vi "read.vi"() -> ()   [LabVIEW 2013]
uses:
  <vilib>/addons/database/Connection.llb/DB Tools Open Connec (Path).vi
  <vilib>/addons/database/_DB Variant To Data/Database Variant To Data.xnode
  <vilib>/addons/database/NI_Database_API.lvlib
panel:
  out "data 3":dbl[](array[numeric])
  out "size(s)":i32
  out "values":variant[](array[variant])
  out "names":string[](array[string])
  out "type string":i16[](array[numeric])
  out "data 2":dbl[](array[numeric])
  out "Waveform Graph":dbl[](graph)
  out "data":variant[][](array[variant])
  out "error out":errorcluster
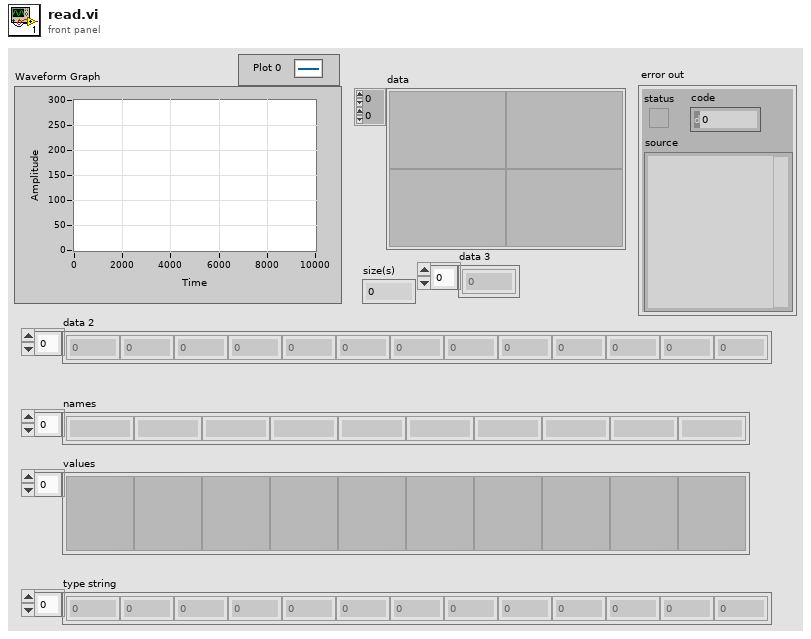
[diagram p1: front panel]
types:
  T1 = typedef "NI_Database_API.lvlib/Conn ObjectReference.ctl" = refnum<k1>
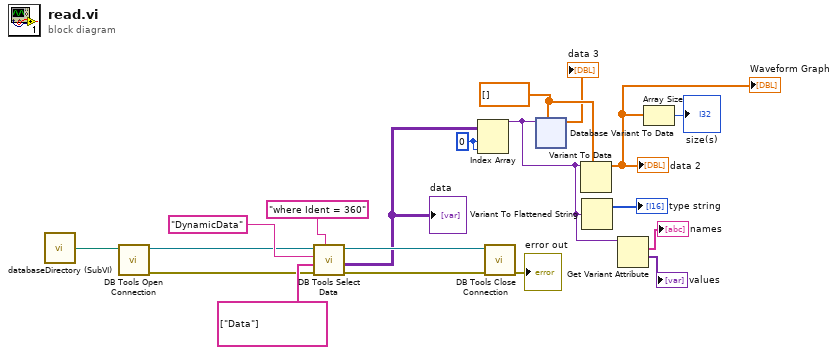
[diagram p0: block diagram]
diagram:
  w8 = dbl[] []
  w9 = 0 ("index")
  n1 = call "databaseDirectory (SubVI).vi"() -> ("Application Directory"=w14:path)  [unwired: 1 in]
  n2 = call-poly <vilib>:"DB Tools Open Connection.vi"("connection information"=w14) -> ("error out"=w13:errorcluster, "connection reference"=w12:T1)  [unwired: 7 in]
  n3 = call <vilib>:"DB Tools Select Data.vi"("condition"="where Ident = 360", "error in (no error)"=w13, "columns"=string[] ["Data"], "table"="DynamicData", "connection reference"=w12) -> ("error out"=w16:errorcluster, "data"=w10:variant[][], "connection reference out"=w17:T1)  [unwired: 1 in]
  "data" <- w10
  n4 = Index Array(array=w10, index (row)=w9, index (col)=w9) -> (element=w6:variant)
  n5 = call <vilib>:"DB Tools Close Connection.vi"("error in (no error)"=w16, "connection reference"=w17) -> ("error out"=→"error out":errorcluster)  [unwired: 5 in]
  n6 = xnode "Database Variant To Data"("database variant"=w6, "type"=w8) -> ("data"=→"data 3":dbl[])  [unwired: 1 in, 1 out]
  n7 = Variant To Data(type=w8, Variant=w6) -> (data=w1:dbl[])  [unwired: 1 in, 1 out]
  "Waveform Graph" <- w1
  "data 2" <- w1
  n8 = Variant To Flattened String(Variant=w6) -> (1:→"type string":i16[])  [unwired: 1 out]
  n9 = Get Variant Attribute(Variant=w6) -> (names=→"names":string[], values=→"values":variant[])  [unwired: 3 in, 2 out]
  n10 = Array Size(array=w1) -> (size(s)=→"size(s)":i32)
